vi "Reaction_space.vi"(8 "error in":errorcluster, 11 "Input cluster":T1) -> (0 "error out":errorcluster, 3 "Ouptut cluster":T1)   [LabVIEW 2020]
uses:
  controls/StateMachineVariables.ctl
  <vilib>/vision/Avi.llb/IMAQ AVI2 Refnum.ctl
  <vilib>/userDefined/High Color/IMAQdx.ctl
  <vilib>/vision/Deep Learning.llb/IMAQ DL Model Refnum.ctl
  <vilib>/vision/Image Controls.llb/IMAQ Image.ctl
panel:
  out "Time to react":string
  out "Speed":dbl format="%#_6p km/h"
  out "Reaction space":cluster{dbl[], dbl[]}[](graph)
  out "clothoid end angle":dbl
  out "clothoid end distance":dbl
  in  "ds":dbl
  out "Clothoid parameter":dbl
  out "Clothoid length":dbl
  out "Max curve radius":dbl
  out "Braking distance":dbl
  in  "Friction coefficient":dbl
  out "Car speed m/s":dbl
  in  "Car speed km/h":dbl
  in  "Y limit":dbl
  in  "Car response time":dbl
  in  "Reaction time":dbl
  in  "Car width":dbl
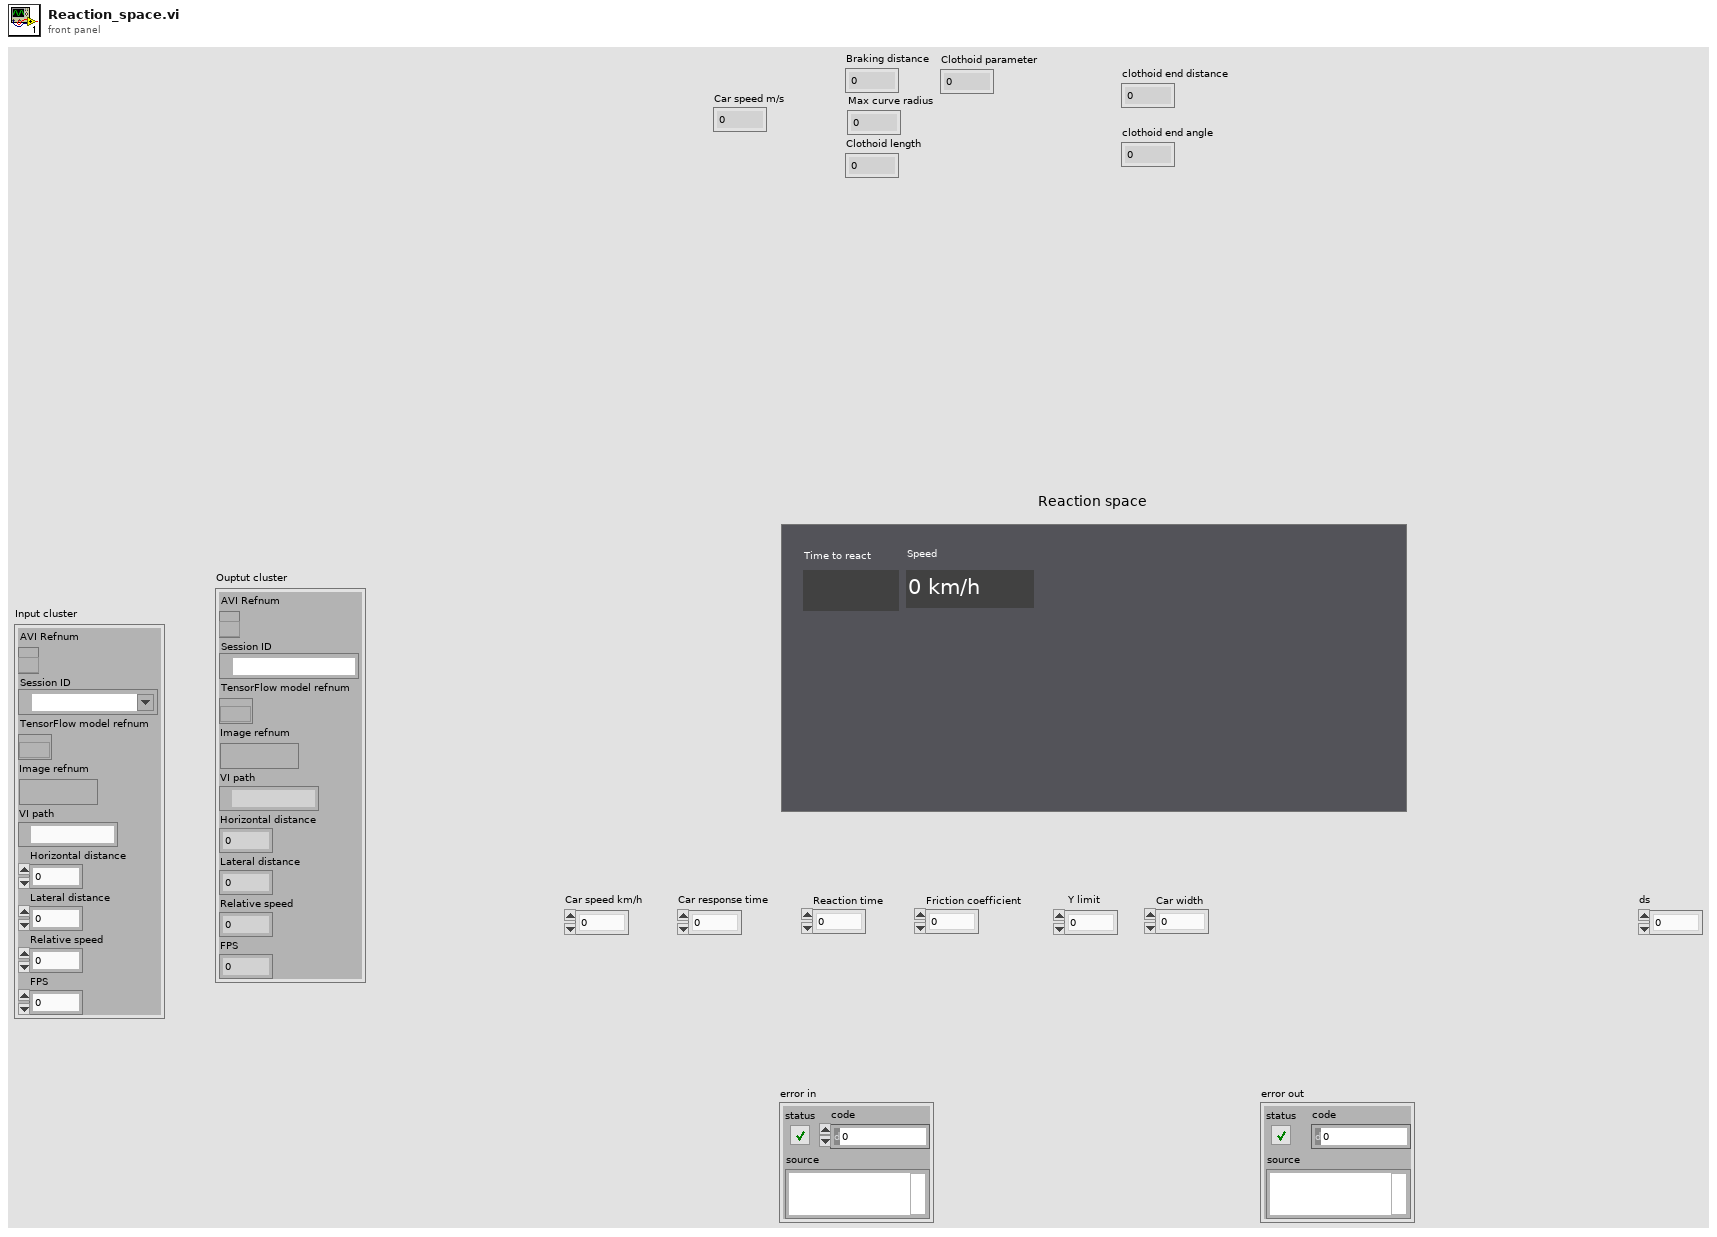
[diagram p1: front panel]
types:
  T1 = typedef "StateMachineVariables.ctl" = cluster{"AVI Refnum":T2, "Session ID":T3, "TensorFlow model refnum":T4, "Image refnum":T5, "VI path":path, "Horizontal distance":dbl, "Lateral distance":dbl, "Relative speed":dbl, "FPS":dbl}
  T2 = typedef "IMAQ AVI2 Refnum.ctl" = refnum<k20>
  T3 = typedef "IMAQdx.ctl" = refnum<k21>
  T4 = typedef "IMAQ DL Model Refnum.ctl" = refnum<k20>
  T5 = typedef "IMAQ Image.ctl" = refnum<image>
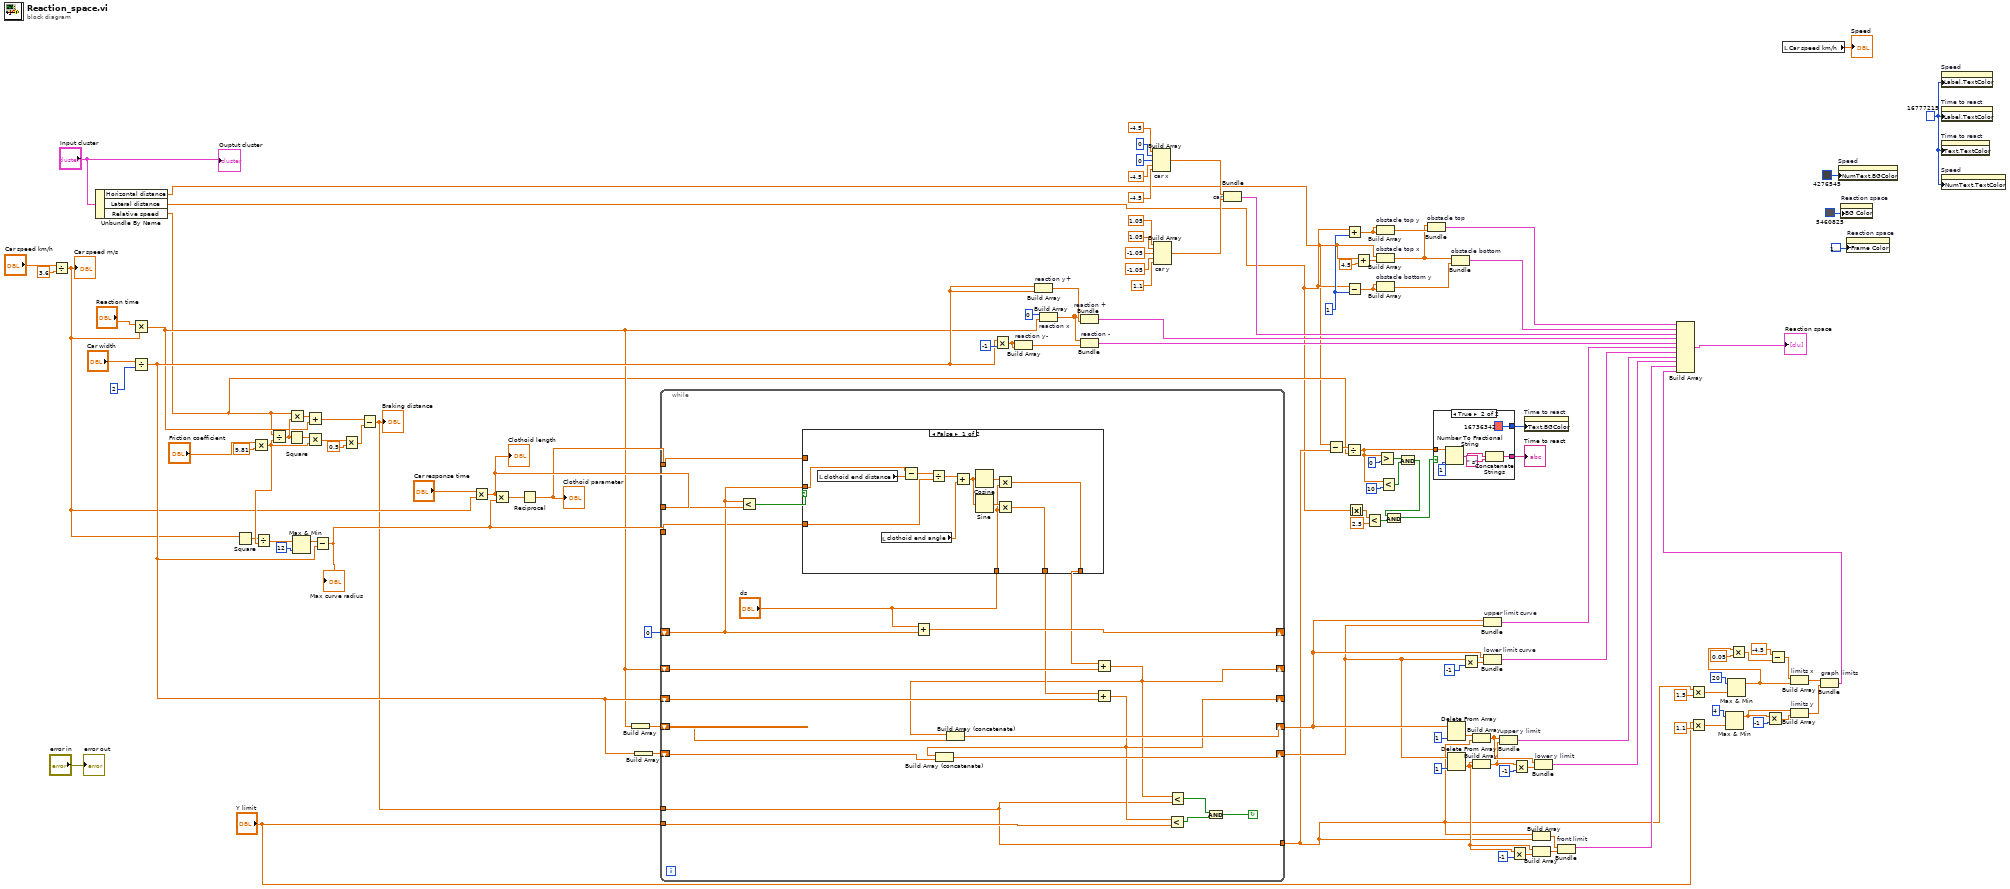
[diagram p0: block diagram]
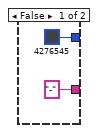
[diagram p2: hidden frame]
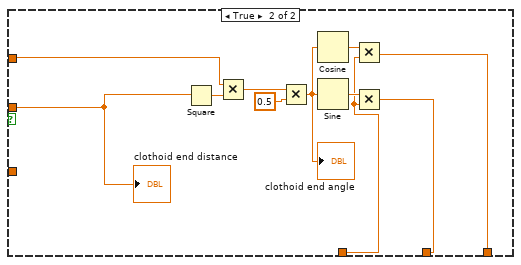
[diagram p3: hidden frame]
diagram:
  w16 = u32 16777215
  w48 = 1
  n1 = Divide(x="Car speed km/h", y=3.6) -> (x/y=w38:dbl)
  "Car speed m/s" <- w38
  n2 = Unbundle By Name("Input cluster") -> ("Horizontal distance"=w1:dbl, "Lateral distance"=w2:dbl, "Relative speed"=w3:dbl)
  n3 = Multiply(x="Reaction time", y=w38) -> (x*y=w35:dbl)
  n4 = Divide(x="Car width", y=2) -> (x/y=w90:dbl)
  n5 = Square(x=w38) -> (x^2=w103:dbl)
  n6 = Multiply(x="Friction coefficient", y=9.81) -> (x*y=w104:dbl)
  n7 = Divide(x=w103, y=w104) -> (x/y=w101:dbl)
  n8 = Divide(x=w3, y=w104) -> (x/y=w109:dbl)
  n9 = Square(x=w109) -> (x^2=w108:dbl)
  n10 = Multiply(x=w3, y=w109) -> (x*y=w111:dbl)
  n11 = Max & Min(x=w101, y=12) -> (max(x,y)=w102:dbl)  [unwired: 1 out]
  n12 = Add(x=w111, y=w35) -> (x+y=w110:dbl)
  n13 = Multiply(x=w108, y=w104) -> (x*y=w107:dbl)
  n14 = Subtract(x=w102, y=w90) -> (x-y=w37:dbl)
  "Max curve radius" <- w37
  n15 = Multiply(x=w107, y=0.5) -> (x*y=w105:dbl)
  n16 = Subtract(x=w110, y=w105) -> (x-y=w36:dbl)
  "Braking distance" <- w36
  n17 = Multiply(x="Car response time", y=w38) -> (x*y=w95:dbl)
  "Clothoid length" <- w95
  n18 = Multiply(x=w95, y=w37) -> (x*y=w98:dbl)
  n19 = Reciprocal(x=w98) -> (1/x=w39:dbl)
  "Clothoid parameter" <- w39
  n20 = Build Array(w35) -> (w92:dbl[])
  n21 = Build Array(w90) -> (w91:dbl[])
  n22 = while "s" {
    shift-right: [w131] -> _
    shift-left: w35 -> [w144]
    shift-right: [w130] -> _
    shift-left: w90 -> [w145]
    shift-right: [w143] -> _
    shift-left: 0 -> [w137]
    tunnel: w95 -> [w142]
    tunnel: w37 -> [w136]
    shift-right: [w132] -> w86
    shift-left: w91 -> [w133]
    shift-right: [w134] -> w89
    shift-left: w92 -> [w135]
    tunnel: w39 -> [w129]
    tunnel: "Y limit" -> [w128]
    tunnel: [w127] -> w12
    tunnel: w36 -> [w127]
    stop <- w146 continue-if-true
    n23 = Less?(x=w137, y=w142) -> (x < y?=w141:bool)
    n24 = case shown="False" w141 {
      tunnel: w137 -> [w160 w162]
      tunnel: "ds" -> [w151 w166]
      tunnel: [w150 w165] -> w139
      tunnel: [w149 w164] -> w138
      tunnel: w136 -> [w157 _]
      tunnel: w129 -> [_ w161]
      frame False {
        n25 = local read "clothoid end distance"() -> (w159:dbl)
        n26 = local read "clothoid end angle"() -> (w156:dbl)
        n27 = Subtract(x=w160, y=w159) -> (x-y=w158:dbl)
        n28 = Divide(x=w158, y=w157) -> (x/y=w155:dbl)
        n29 = Add(x=w155, y=w156) -> (x+y=w154:dbl)
        n30 = Cosine(x=w154) -> (cos(x)=w153:dbl)
        n31 = Sine(x=w154) -> (sin(x)=w152:dbl)
        n32 = Multiply(x=w153, y=w151) -> (x*y=w150:dbl)
        n33 = Multiply(x=w152, y=w151) -> (x*y=w149:dbl)
      }
      frame True {
        n34 = Square(x=w162) -> (x^2=w171:dbl)
        n35 = Multiply(x=w161, y=w171) -> (x*y=w170:dbl)
        n36 = Multiply(x=w170, y=0.5) -> (x*y=w163:dbl)
        "clothoid end angle" <- w163
        n37 = Cosine(x=w163) -> (cos(x)=w168:dbl)
        n38 = Sine(x=w163) -> (sin(x)=w167:dbl)
        n39 = Multiply(x=w168, y=w166) -> (x*y=w165:dbl)
        n40 = Multiply(x=w167, y=w166) -> (x*y=w164:dbl)
        "clothoid end distance" <- w162
      }
    }
    n41 = Add(x="ds", y=w137) -> (x+y=w143:dbl)
    n42 = Add(x=w139, y=w144) -> (x+y=w131:dbl)
    n43 = Build Array (concatenate)(w131, w135) -> (w134:dbl[])
    n44 = Add(x=w138, y=w145) -> (x+y=w130:dbl)
    n45 = Build Array (concatenate)(w130, w133) -> (w132:dbl[])
    n46 = Less?(x=w130, y=w128) -> (x < y?=w148:bool)
    n47 = Less?(x=w131, y=w127) -> (x < y?=w147:bool)
    n48 = And(x=w147, y=w148) -> (x .and. y?=w146:bool)
  }
  n49 = Multiply(x=w90, y=-1) -> (x*y=w122:dbl)
  n50 = Build Array "reaction y-"(w122, w122) -> (w120:dbl[])
  n51 = Build Array "reaction y+"(w90, w90) -> (w121:dbl[])
  n52 = Build Array "reaction x"(0, w35) -> (w119:dbl[])
  n53 = Bundle "reaction +"(w119, w121) -> (w118:cluster{dbl[], dbl[]})  [unwired: 1 in]
  n54 = Bundle "reaction -"(w119, w120) -> (w117:cluster{dbl[], dbl[]})  [unwired: 1 in]
  n55 = Build Array "car x"(-4.5, 0, 0, -4.5, -4.5) -> (w64:dbl[])
  n56 = Build Array "car y"(1.05, 1.05, -1.05, -1.05, 1.1) -> (w63:dbl[])
  n57 = Bundle "car"(w64, w63) -> (w62:cluster{dbl[], dbl[]})  [unwired: 1 in]
  n58 = Subtract(x=w1, y=w12) -> (x-y=w22:dbl)
  n59 = Divide(x=w22, y=w3) -> (x/y=w17:dbl)
  n60 = Add(x=w2, y=w48) -> (x+y=w56:dbl)
  n61 = Subtract(x=w2, y=w48) -> (x-y=w52:dbl)
  n62 = Absolute Value(x=w2) -> (abs(x)=w10:dbl)
  n63 = Add(x=w1, y=4.5) -> (x+y=w58:dbl)
  n64 = Less?(x=w10, y=2.5) -> (x < y?=w6:bool)
  n65 = Build Array "obstacle top y"(w56, w56) -> (w57:dbl[])
  n66 = Build Array "obstacle top x"(w1, w58) -> (w53:dbl[])
  n67 = Build Array "obstacle bottom y"(w52, w52) -> (w55:dbl[])
  n68 = Greater?(x=w17, y=0) -> (0:w18:bool)
  n69 = Less?(x=w17, y=10) -> (x < y?=w19:bool)
  n70 = And(x=w18, y=w19) -> (x .and. y?=w7:bool)
  n71 = And(x=w7, y=w6) -> (x .and. y?=w8:bool)
  n72 = Bundle "obstacle top"(w53, w57) -> (w54:cluster{dbl[], dbl[]})  [unwired: 1 in]
  n73 = case shown="True" w8 {
    tunnel: ["-" w179] -> w15
    tunnel: w17 -> [_ w176]
    tunnel: [u32 4276545 u32 16736342] -> w14
    frame False {
    }
    frame True {
      n74 = Number To Fractional String(number=w176, precision (6)=1) -> (F-format string=w175:string)  [unwired: 2 in]
      n75 = Concatenate Strings(w175, " s") -> (w179:string)
    }
  }
  "Time to react" <- w15
  n76 = Delete From Array(array=w89, index=1) -> (deleted portion=w13:dbl)  [unwired: 1 in, 1 out]
  n77 = Delete From Array(array=w86, index=1) -> (deleted portion=w76:dbl)  [unwired: 1 in, 1 out]
  n78 = Bundle "obstacle bottom"(w53, w55) -> (w51:cluster{dbl[], dbl[]})  [unwired: 1 in]
  n79 = Multiply(x=w86, y=-1) -> (x*y=w94:dbl[])
  n80 = Build Array(w13, w12) -> (w84:dbl[])
  n81 = Build Array(w76, w76) -> (w81:dbl[])
  n82 = Bundle "upper limit curve"(w89, w86) -> (w97:cluster{dbl[], dbl[]})  [unwired: 1 in]
  n83 = Bundle "lower limit curve"(w89, w94) -> (w93:cluster{dbl[], dbl[]})  [unwired: 1 in]
  n84 = Bundle "upper y limit"(w84, w81) -> (w80:cluster{dbl[], dbl[]})  [unwired: 1 in]
  n85 = Multiply(x=w76, y=-1) -> (x*y=w78:dbl)
  n86 = Multiply(x=w81, y=-1) -> (x*y=w82:dbl[])
  n87 = property on="Time to react" class="Str"("Text.BGColor"=w14) -> ()  [unwired: 2 in, 2 out]
  n88 = Build Array(w12, w12) -> (w75:dbl[])
  n89 = Build Array(w76, w78) -> (w74:dbl[])
  n90 = Bundle "lower y limit"(w84, w82) -> (w79:cluster{dbl[], dbl[]})  [unwired: 1 in]
  n91 = Bundle "front limit"(w75, w74) -> (w73:cluster{dbl[], dbl[]})  [unwired: 1 in]
  n92 = Multiply(x=w12, y=1.5) -> (x*y=w40:dbl)
  n93 = Multiply(x="Y limit", y=1.1) -> (x*y=w30:dbl)
  n94 = Max & Min(x=4, y=w30) -> (max(x,y)=w27:dbl)  [unwired: 1 out]
  n95 = Max & Min(x=20, y=w40) -> (max(x,y)=w11:dbl)  [unwired: 1 out]
  n96 = Multiply(x=w11, y=0.05) -> (x*y=w43:dbl)
  n97 = Multiply(x=w27, y=-1) -> (x*y=w26:dbl)
  n98 = Subtract(x=-4.5, y=w43) -> (x-y=w33:dbl)
  n99 = local read "Car speed km/h"() -> (→"Speed":dbl)
  n100 = Build Array "limits x"(w33, w11) -> (w24:dbl[])
  n101 = Build Array "limits y"(w27, w26) -> (w25:dbl[])
  n102 = Bundle "graph limits"(w24, w25) -> (w23:cluster{dbl[], dbl[]})  [unwired: 1 in]
  n103 = Build Array(w54, w51, w62, w118, w117, w97, w93, w80, w79, w73, w23) -> (→"Reaction space":cluster{dbl[], dbl[]}[])
  n104 = property on="Speed" class="DigNum (strict)"("NumText.BGColor"=u32 4276545) -> ()  [unwired: 2 in, 2 out]
  n105 = property on="Reaction space" class="XYGraph (strict)"("BG Color"=u32 5460825) -> ()  [unwired: 2 in, 2 out]
  n106 = property on="Reaction space" class="XYGraph (strict)"("Frame Color"=u32 16777216) -> ()  [unwired: 2 in, 2 out]
  n107 = property on="Speed" class="DigNum (strict)"("Label.TextColor"=w16) -> ()  [unwired: 2 in, 2 out]
  n108 = property on="Time to react" class="Str"("Label.TextColor"=w16) -> ()  [unwired: 2 in, 2 out]
  n109 = property on="Time to react" class="Str"("Text.TextColor"=w16) -> ()  [unwired: 2 in, 2 out]
  n110 = property on="Speed" class="DigNum (strict)"("NumText.TextColor"=w16) -> ()  [unwired: 2 in, 2 out]
  "error out" <- "error in"
  "Ouptut cluster" <- "Input cluster"
